vi "Webpublish.vi"() -> ()   [LabVIEW 2011]
panel:
  in  "stop":bool
  out "Numeric":dbl
  in  "Boolean":bool
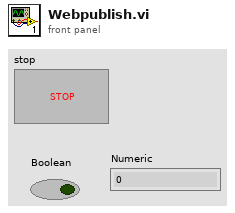
[diagram p1: front panel]
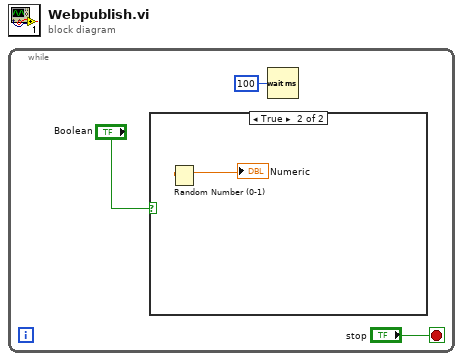
[diagram p0: block diagram]
diagram:
  n1 = while {
    stop <- "stop" stop-if-true
    n2 = case shown="True" "Boolean" {
      frame False {
      }
      frame True {
        n3 = Random Number (0-1)() -> (number: 0 to 1=→"Numeric":dbl)
      }
    }
    n4 = Wait (ms)(milliseconds to wait=u32 100) -> ()  [unwired: 1 out]
  }
